vi "Get Item by Index.vi"(8 "error in (no error)":errorcluster caption="错误输入（无错误）", 10 "index":i32, 11 "ArrayListClass 输入":refnum<class "ArrayListClass.lvclass"> caption="DNL_LabVIEW Object in") -> (0 "error out":errorcluster caption="错误输出", 2 "Value":variant, 3 "ArrayListClass 输出":refnum<class "ArrayListClass.lvclass"> caption="DNL_LabVIEW Object out")   [LabVIEW 2012, in "ArrayListClass.lvclass"]
uses:
  ArrayListClass.lvclass
  ArrayListClass.lvclass/ArrayListClass.ctl
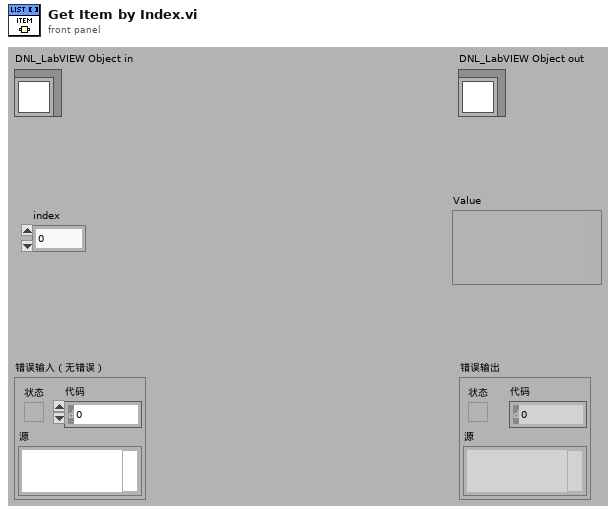
[diagram p1: front panel]
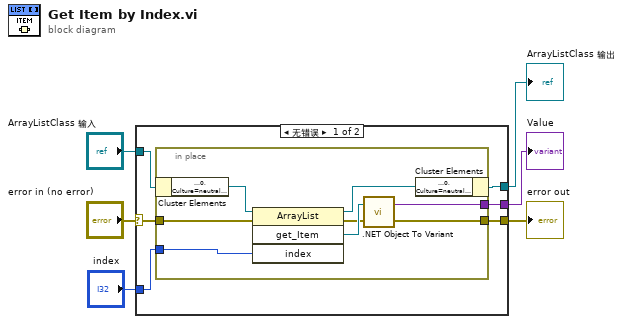
[diagram p0: block diagram]
diagram:
  n1 = case shown="无错误" "error in (no error)" {
    selector: "error in (no error)" -> [w10 w22]
    tunnel: [w9 w22] -> w5
    tunnel: [w11 w21] -> w3
    tunnel: "ArrayListClass 输入" -> [w12 w21]
    tunnel: "index" -> [w8 _]
    tunnel: [w7 _] -> w1
    frame No Error {
      n2 = in-place {
        in-place-border: w10 -> [w18]
        in-place-border: [w14] -> w9
        in-place-border: w8 -> [w17]
        in-place-border: [w13] -> w7
        n3 = in-place-cluster #1(w12) -> ("ArrayList"=w20:refnum<k24>)
        n4 = invoke class="ArrayList" method="get_Item"(reference=w20, error in=w18, "index"=w17) -> (reference out=w19:refnum<k24>, error out=w15:errorcluster, "get_Item"=w16:refnum<k24>)  [unwired: 1 in, 1 out]
        n5 = call <vilib>:".NET Object To Variant.vi"("error in (no error)"=w15, ".NET object"=w16) -> ("error out"=w14:errorcluster, "variant"=w13:variant)
        n6 = in-place-cluster #1("ArrayList"=w19) -> (w11:refnum<class "ArrayListClass.lvclass">)
      }
    }
    frame Error {
    }
  }
  "error out" <- w5
  "ArrayListClass 输出" <- w3
  "Value" <- w1
